vi "Stop.vi"(8 "error in (no error)":errorcluster, 11 "Scope PXI in":refnum<class "Scope PXI.lvclass">) -> (0 "error out":errorcluster, 3 "Scope PXI out":refnum<class "Scope PXI.lvclass">)   [LabVIEW 2023, in "Scope.lvlib" / "Scope PXI.lvlib" / "Scope PXI.lvclass"]
uses:
  Scope PXI.lvclass
  <vilib>/Utility/error.llb/Error Cluster From Error Code.vi
  <vilib>/ErrorRing/Error Ring.xnode
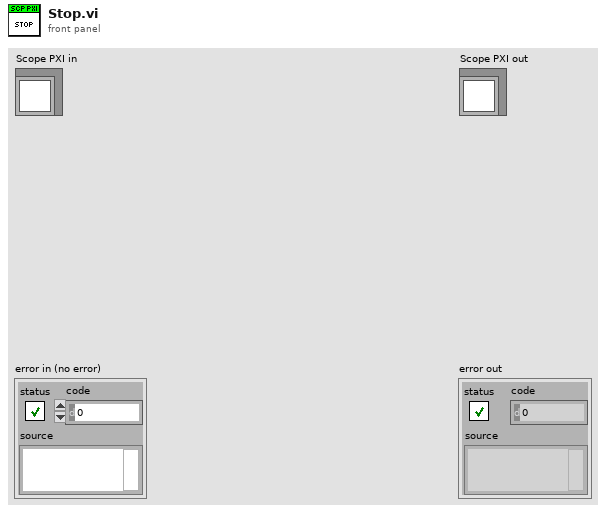
[diagram p1: front panel]
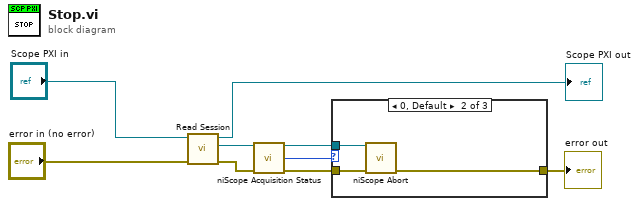
[diagram p0: block diagram]
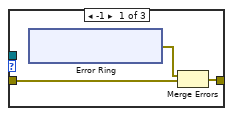
[diagram p2: hidden frame]
diagram:
  n1 = call "Read Session.vi"("error in (no error)"="error in (no error)", "Scope PXI in"="Scope PXI in") -> ("error out"=w5:errorcluster, "session"=w3:refnum<k15>, "Scope PXI out"=→"Scope PXI out":refnum<class "Scope PXI.lvclass">)  [unwired: 7 in]
  n2 = call <instrlib>:"niScope Acquisition Status.vi"("instrument handle"=w3, "error in"=w5) -> ("instrument handle out"=w2:refnum<k15>, "acquisition status"=w1:i32, "error out"=w4:errorcluster)  [unwired: 11 in]
  n3 = case shown="0, Default" w1 {
    tunnel: [w12 w20 w21] -> w7
    tunnel: w4 -> [w10 w19 w21]
    tunnel: w2 -> [_ w18 _]
    frame -1 {
      n4 = xnode "Error Ring"() -> ("error out"=w11:errorcluster)
      n5 = Merge Errors(w11, w10) -> (w12:errorcluster)
    }
    frame 0, Default {
      n6 = call <instrlib>:"niScope Abort.vi"("instrument handle"=w18, "error in"=w19) -> ("error out"=w20:errorcluster)  [unwired: 12 in, 1 out]
    }
    frame 1 {
    }
  }
  "error out" <- w7
